vi "Connect Seq List View.vi"(8 "error in (no error)":errorcluster, 11 "teststand-api in":refnum<class "teststand-api.lvclass">) -> (0 "error out":errorcluster, 3 "teststand-api out":refnum<class "teststand-api.lvclass">)   [LabVIEW 2014, in "teststand-api.lvlib" / "teststand-api.lvclass"]
uses:
  teststand-api.lvclass
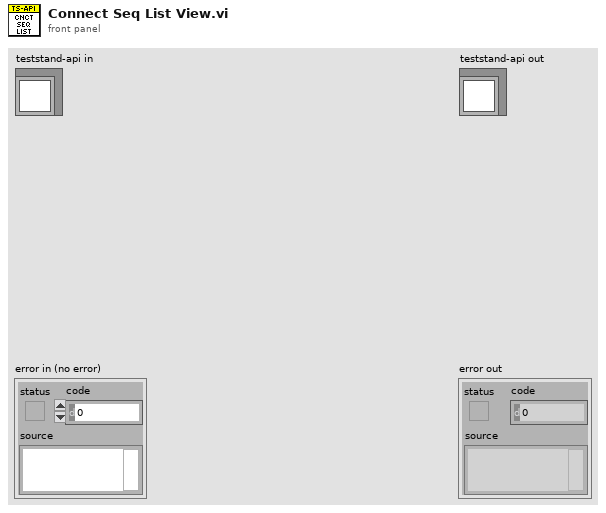
[diagram p1: front panel]
types:
  T1 = typedef "teststand-api.lvlib/teststand-api.lvclass/TS Controls Argument--cluster.ctl" = cluster{"Execution View":refnum<k7>, "Sequence View":refnum<k7>, "Report View":refnum<k7>, "Seq List":refnum<k7>}
  T2 = typedef "teststand-api.lvlib/teststand-api.lvclass/Manager Controls Argument--cluster.ctl" = cluster{"App Manager":refnum<k7>, "Seq Manager":refnum<k7>, "Exec Manager":refnum<k7>}
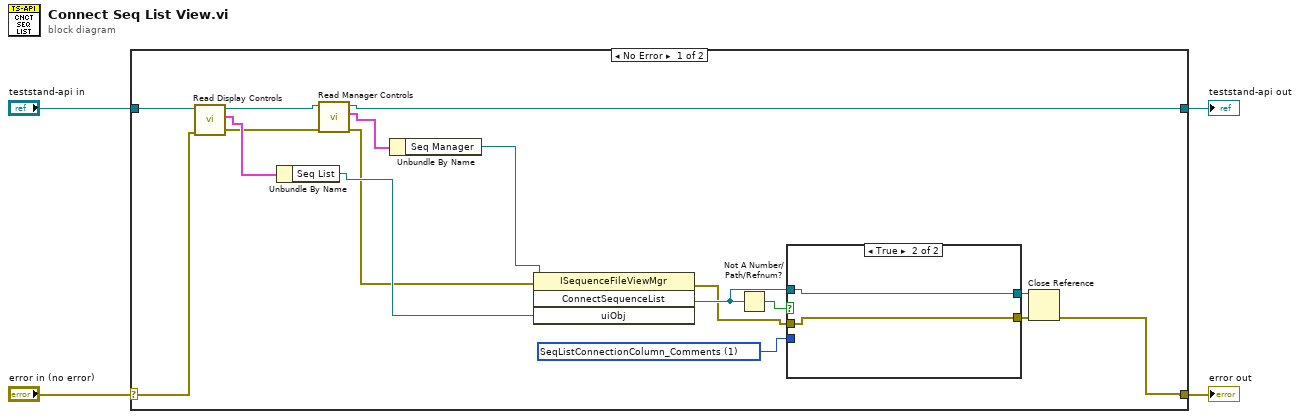
[diagram p0: block diagram]
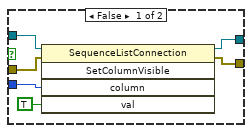
[diagram p2: hidden frame]
diagram:
  n1 = case shown="No Error" "error in (no error)" {
    selector: "error in (no error)" -> [w14 w31]
    tunnel: [w12 w31] -> w3
    tunnel: [w21 w30] -> w1
    tunnel: "teststand-api in" -> [w18 w30]
    frame No Error {
      w8 = 1 items=["SeqListConnectionColumn_Label", "SeqListConnectionColumn_Comments", "SeqListConnectionColumn_Requirements"] ("column")
      n2 = call-dynamic "Read Display Controls.vi"("error in (no error)"=w14, "teststand-api in"=w18) -> ("error out"=w15:errorcluster, "Visible Controls"=w16:T1, "teststand-api out"=w17:refnum<class "teststand-api.lvclass">)  [unwired: 7 in]
      n3 = Unbundle By Name(w16) -> ("Seq List"=w13:refnum<k7>)
      n4 = call-dynamic "Read Manager Controls.vi"("error in (no error)"=w15, "teststand-api in"=w17) -> ("error out"=w11:errorcluster, "Manager Controls"=w20:T2, "teststand-api out"=w21:refnum<class "teststand-api.lvclass">)  [unwired: 7 in]
      n5 = Unbundle By Name(w20) -> ("Seq Manager"=w19:refnum<k7>)
      n6 = invoke class="ISequenceFileViewMgr" method="ConnectSequenceList"(reference=w19, error in=w11, "uiObj"=w13) -> (error out=w5:errorcluster, "ConnectSequenceList"=w9:refnum<k7>)  [unwired: 1 in, 2 out]
      n7 = Not A Number/Path/Refnum?(number/path/refnum=w9) -> (NaN/Path/Refnum?=w10:bool)
      n8 = case shown="True" w10 {
        tunnel: w9 -> [w27 w29]
        tunnel: w8 -> [w25 _]
        tunnel: [w24 w28] -> w7
        tunnel: [w23 w29] -> w6
        tunnel: w5 -> [w22 w28]
        frame False {
          n9 = invoke class="SequenceListConnection" method="SetColumnVisible"(reference=w27, error in=w22, "column"=w25, "val"=TRUE) -> (reference out=w23:refnum<k7>, error out=w24:errorcluster)  [unwired: 1 in, 3 out]
        }
        frame True {
        }
      }
      n10 = Close Reference(reference=w6, error in (no error)=w7) -> (error out=w12:errorcluster)
    }
    frame Error {
    }
  }
  "error out" <- w3
  "teststand-api out" <- w1
